vi "Get (I16).vi"(8 "error in":errorcluster, 11 "Value in":refnum<class "Value.lvclass">) -> (0 "error out":errorcluster, 1 "Defined?":bool, 2 "Value":i16, 3 "Value out":refnum<class "Value.lvclass">)   [LabVIEW 2024, in "Electronic Datasheet.lvlib" / "Value.lvclass"]
uses:
  Value.lvclass
  Value.lvclass/Value.ctl
  Electronic Datasheet.lvlib
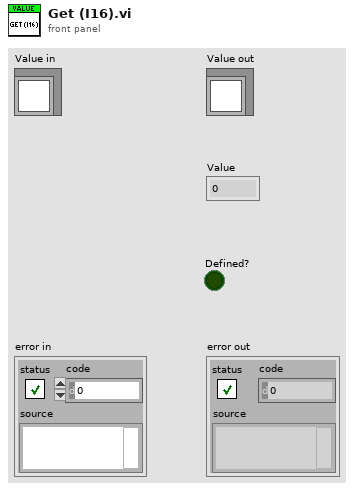
[diagram p1: front panel]
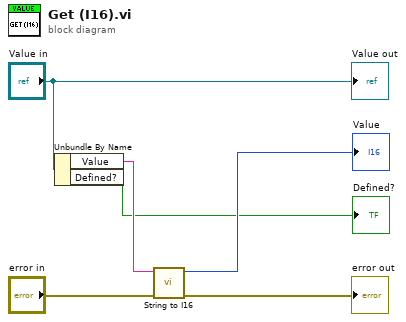
[diagram p0: block diagram]
diagram:
  n1 = Unbundle By Name("Value in") -> ("Value"=w5:string, "Defined?"=→"Defined?":bool)
  n2 = call "String to I16.vi"("error in"="error in", "String"=w5) -> ("error out"=→"error out":errorcluster, "I16"=→"Value":i16)  [unwired: 8 in]
  "Value out" <- "Value in"
